vi "Robot Global Data.vi"() -> ()   [LabVIEW 2013]
doc: "This global VI can contain as many global variables as you need. Place a control on the panel, give it a good name. To read or write to it from a VI, drag the icon to the diagram of that VI. You can also drag from the project. Click on the node to change which global you access. You shouldn't have multiple locations writing to a global or it will cause a race-condition."
uses:
  <vilib>/Rock Robotics/WPI/Camera/WPI_CameraImageSize.ctl
  <vilib>/Rock Robotics/WPI/DriverStation/WPI_DriverStationRobotMode2.ctl
panel:
  in  "Header":dbl=2.2320031374200004
  in  "Teleop Run Time":dbl=57.141
  out "Shooter at Speed":bool
  in  "Desired Shooter Speed":dbl=15.0
  in  "Shooter Index Offset":i32=10
  in  "Shooter Angles":dbl[](array[numeric])=[2.6, 3.45, 3.45, 3.45, 3.45]
  in  "Shooter Speeds":dbl[](array[numeric])=[45.0, 45.0, 45.0, 45.0, 45.0]
  in  "Lifter Position":i8=3
  in  "Shoot Distance":i32=10 min=0 max=54 step=1
  out "Keep Gate Open":bool
  out "Target Info":T1(array[cluster])
  in  "Robot Mode":T2=enum."Finish"
  in  "LED toggle rate (ms)":u32=100
  in  "image size":T3=enum."320x240"
  in  "Enable Vision":bool
  # "10 ft"
  # "11 ft"
  # "12 ft"
  # "13 ft"
  # "14 ft"
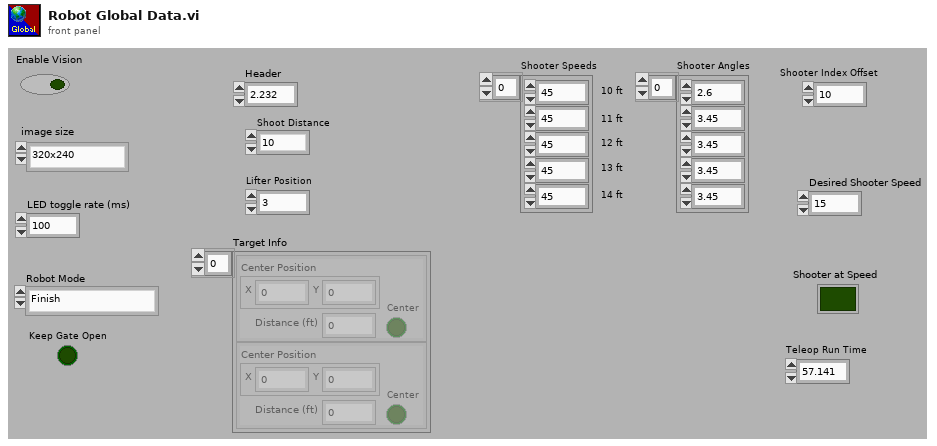
[diagram p1: front panel]
types:
  T1 = cluster{"Center Position":cluster{"X":dbl, "Y":dbl}, "Distance (ft)":dbl, "Center":bool}[]
  T2 = typedef "WPI_DriverStationRobotMode2.ctl" = enum16{"Autonomous Disabled", "Autonomous Enabled", "Teleop Disabled", "Teleop Enabled", "Timeout", "Finish", "Test Disabled", "Test Enabled"}
  T3 = typedef "WPI_CameraImageSize.ctl" = enum16{"640x480", "320x240", "160x120"}
diagram:
